vi "Create Sensor.vi"(4 "Scale Params":dbl[](array[numeric]), 6 "Scale Type":T1, 8 "error in (no error)":errorcluster, 10 "Sensor ID":string, 11 "SensorList in":refnum<class "SensorList.lvclass">) -> (0 "error out":errorcluster, 3 "SensorList out":refnum<class "SensorList.lvclass">)   [LabVIEW 2020, in "VolatusConfig.lvlib" / "SensorList.lvclass"]
uses:
  SensorList.lvclass
  SensorList.lvclass/SensorList.ctl
  VolatusConfigElement/VolatusConfigElement.lvclass
  lv-cdm/CDM-Config/Config Element/Config Element.lvclass
  Sensor/Sensor Config.lvclass
  C:/dev/lv20CE/relink/lv-volatus/VolatusConfig/VolatusConfigElement/VolatusConfigElement.lvclass
  C:/dev/lv20CE/relink/lv-volatus/VolatusConfig/SensorList/SensorList.lvclass
  Scale Type.ctl
  VolatusConfig.lvlib
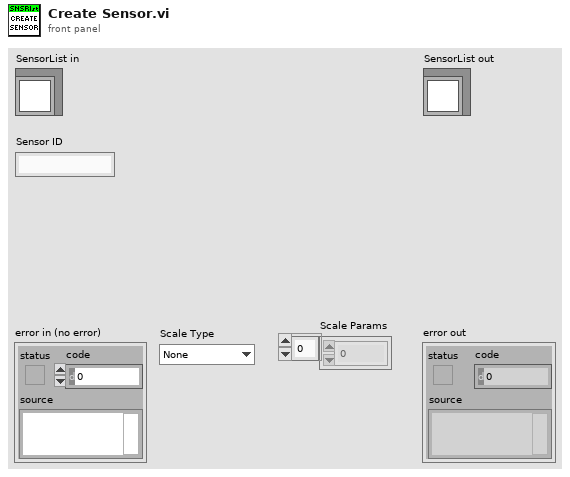
[diagram p1: front panel]
types:
  T1 = typedef "VolatusConfig.lvlib/Scale Type.ctl" = enum16{"None", "Sensor", "Polynomial", "Threshold", "Invert Bool", "Exponential"}
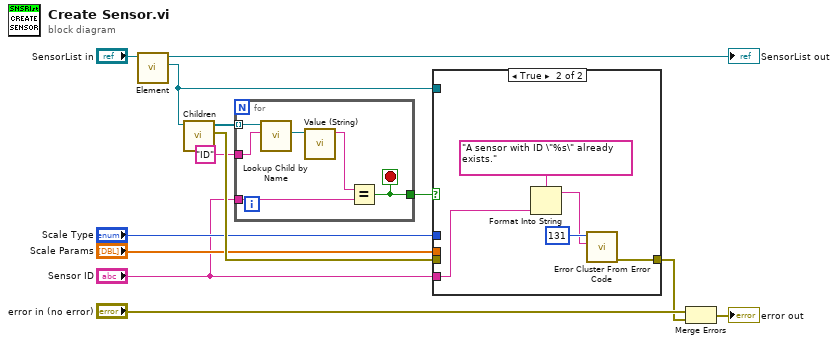
[diagram p0: block diagram]
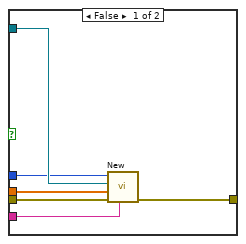
[diagram p2: hidden frame]
diagram:
  n1 = call "Element.vi"("VolatusConfigElement in"="SensorList in") -> ("Element"=w5:refnum<class "Config Element.lvclass">, "VolatusConfigElement out"=→"SensorList out":refnum<class "SensorList.lvclass">)  [unwired: 9 in]
  n2 = call "Children.vi"("Config Element in"=w5) -> ("error out"=w13:errorcluster, "Elements"=w4:refnum<class "Config Element.lvclass">[])  [unwired: 9 in]
  n3 = for {
    tunnel: w4 -> [w19] mode=indexing
    tunnel: "ID" -> [w18]
    tunnel: [w15] -> w8
    tunnel: "Sensor ID" -> [w14]
    stop <- w15 stop-if-true
    n4 = call "Lookup Child by Name.vi"("Name"=w18, "Config Element in"=w19) -> ("Child"=w17:refnum<class "Config Element.lvclass">)  [unwired: 6 in, 3 out]
    n5 = call "Value (String).vi"("Config Element in"=w17) -> ("String Value"=w16:string)  [unwired: 9 in, 1 out]
    n6 = Equal?(x=w16, y=w14) -> (x = y?=w15:bool)
  }
  n7 = case shown="True" w8 {
    tunnel: "Sensor ID" -> [w22 w26]
    tunnel: [w20 w27] -> w2
    tunnel: "Scale Type" -> [w24 _]
    tunnel: "Scale Params" -> [w23 _]
    tunnel: w5 -> [w25 _]
    tunnel: w13 -> [w21 _]
    frame False {
      n8 = call "New.vi"("Sensor ID"=w22, "error in (no error)"=w21, "Scale Params"=w23, "Parent"=w25, "Scale Type"=w24) -> ("error out"=w20:errorcluster)  [unwired: 5 in, 1 out]
    }
    frame True {
      n9 = Format Into String(format string="A sensor with ID \"%s\" already exists.", w26) -> (resulting string=w28:string)  [unwired: 2 in, 1 out]
      n10 = call <vilib>:"Error Cluster From Error Code.vi"("error message (\"\")"=w28, "error code (0)"=131) -> ("error out"=w27:errorcluster)  [unwired: 7 in]
    }
  }
  n11 = Merge Errors("error in (no error)", w2) -> (→"error out":errorcluster)
